vi "_Remove Capabilities.vi"(8 "error in (no error)":errorcluster, 10 "Capabilities":string[](array[string]), 11 "NodeDiscovery in":refnum<class "DiscoveryService.lvclass">) -> (0 "error out":errorcluster, 3 "NodeDiscovery out":refnum<class "DiscoveryService.lvclass">)   [LabVIEW 2020, in "Vecto.lvlib" / "DiscoveryService.lvclass"]
uses:
  DiscoveryService.lvclass
  DiscoveryService.lvclass/DiscoveryService.ctl
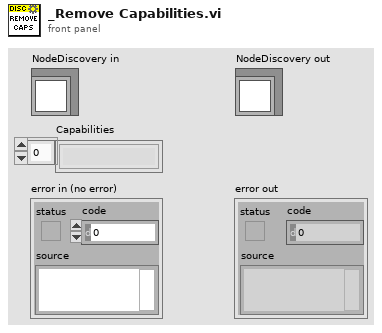
[diagram p1: front panel]
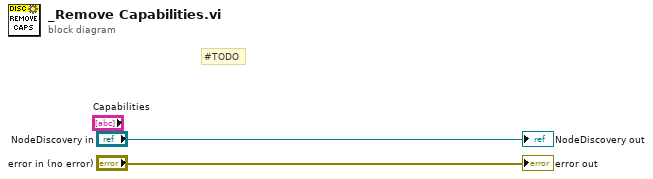
[diagram p0: block diagram]
diagram:
  # "#TODO"
  "error out" <- "error in (no error)"
  "NodeDiscovery out" <- "NodeDiscovery in"
